vi "Filter Files.vi"(1 "Start Time":timestamp, 2 "End Time":timestamp, 5 "filenames in":string[](array[string]), 7 "filesizes (bytes) in":i64[](array[numeric]), 9 "last modificadtion data in":timestamp[](array[timestamp]), 11 "error in":errorcluster) -> (6 "filenames out":string[](array[string]), 8 "filesizes (bytes) out":i64[](array[numeric]), 10 "last modificadtion data out":timestamp[](array[timestamp]), 14 "# of files":i32, 15 "error out":errorcluster)   [LabVIEW 2019]
doc: "Filter Files by data."
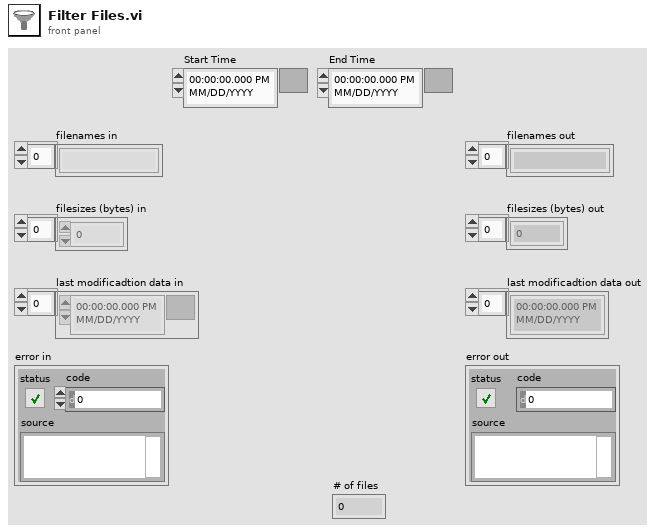
[diagram p1: front panel]
types:
  T1 = typedef "LVDateTimeRec.ctl" = cluster{"fractional second":dbl, "second":i32, "minute":i32, "hour":i32, "day of month":i32, "month":i32, "year":i32, "day of week":i32, "day of year":i32, "DST":i32}
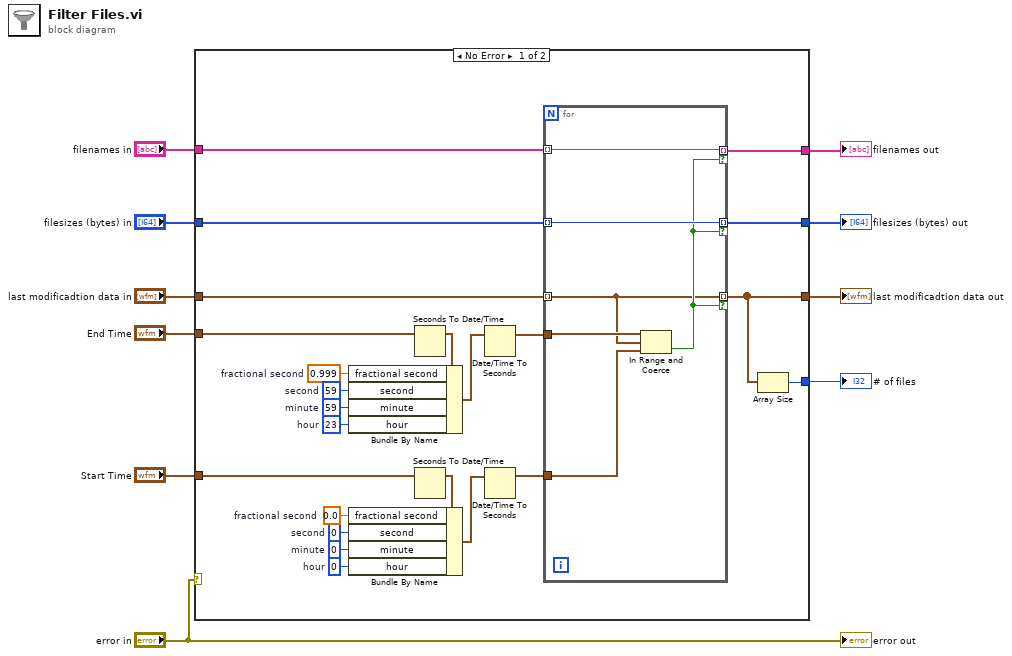
[diagram p0: block diagram]
diagram:
  n1 = case shown="No Error" "error in" {
    tunnel: "filenames in" -> [w33 _]
    tunnel: "filesizes (bytes) in" -> [w32 _]
    tunnel: [w31 _] -> w8
    tunnel: [w30 _] -> w7
    tunnel: "last modificadtion data in" -> [w29 _]
    tunnel: [w28 _] -> w5
    tunnel: [w27 _] -> w4
    tunnel: "Start Time" -> [w20 _]
    tunnel: "End Time" -> [w12 _]
    frame No Error {
      w13 = 23  # hour
      w14 = 59  # minute
      w15 = 59  # second
      w16 = 0.999  # fractional second
      w26 = 0  # hour
      w25 = 0  # minute
      w24 = 0  # second
      w23 = 0.0  # fractional second
      n2 = Seconds To Date/Time(time stamp (now)=w12) -> (date time rec=w17:T1)  [unwired: 1 in]
      n3 = Bundle By Name(cluster=w17, "fractional second"=w16, "second"=w15, "minute"=w14, "hour"=w13) -> (w18:T1)
      n4 = Seconds To Date/Time(time stamp (now)=w20) -> (date time rec=w22:T1)  [unwired: 1 in]
      n5 = Bundle By Name(cluster=w22, "fractional second"=w23, "second"=w24, "minute"=w25, "hour"=w26) -> (w21:T1)
      n6 = Date/Time To Seconds(2:w18) -> (0:w11:timestamp)  [unwired: 1 in]
      n7 = Date/Time To Seconds(2:w21) -> (0:w19:timestamp)  [unwired: 1 in]
      n8 = for {
        tunnel: w33 -> [w39] mode=indexing
        tunnel: [w39] -> w30 mode=indexing if=w35
        tunnel: w32 -> [w38] mode=indexing
        tunnel: [w38] -> w31 mode=indexing if=w35
        tunnel: w29 -> [w34] mode=indexing
        tunnel: [w34] -> w28 mode=indexing if=w35
        tunnel: w19 -> [w37]
        tunnel: w11 -> [w36]
        n9 = In Range and Coerce(upper limit=w36, x=w34, lower limit=w37) -> (In Range?=w35:bool)  [unwired: 1 out]
      }
      n10 = Array Size(array=w28) -> (size(s)=w27:i32)
    }
    frame Error {
    }
  }
  "filenames out" <- w7
  "filesizes (bytes) out" <- w8
  "# of files" <- w4
  "last modificadtion data out" <- w5
  "error out" <- "error in"
